vi "Main.vi"() -> ()   [LabVIEW 2017]
doc: "This Continuous Measurement sample project is based on the Queued Message Handler template.\n\nThe Event Handling Loop generates messages based on user interface actions.\n\nThe Message Handling Loop processes messages generated by the Event Handling Loop, or by other messages. There are also Acquisition and Logging message handling loop subVIs, and a chart updating loop."
uses:
  Settings/Settings.ctl
  Acquisition/Hardware Configuration.ctl
  Acquisition/Signal Type.ctl
  Logging/Logging Configuration.ctl
  controls/UI Data.ctl
  controls/UI State.ctl
  support/Message Queue/Enqueue Message (Single).vi
  support/Message Queue/Enqueue Message (Array).vi
  <vilib>/Utility/error.llb/Error Cluster From Error Code.vi
  <vilib>/ErrorRing/Error Ring.xnode
  Acquisition/Acquisition.lvlib
  Logging/Logging.lvlib
  Settings/Settings.lvlib
  support/User Event - Stop/User Event - Stop.lvlib
  support/Message Queue/Message Queue.lvlib
  Settings/Settings Dialog.vi
panel:
  out "Elapsed time":timestamp
  in  "Start waves":bool
  in  "Initialize wave maker":bool
  in  "Preview wave file":bool
  in  "Wave file":path
  in  "Testing time zero run [s]":dbl
  in  "Testing time [s]":dbl
  in  "Zero run?":bool
  in  "Stop":bool
  in  "Start":bool
  in  "Settings":bool
  out "Status":string
  in  "Exit":bool
  out "Waves preview":waveform(dbl)[](graph)
  out "Data":waveform(dbl)[](graph)
  # "Continuous Measurement Data Logger"
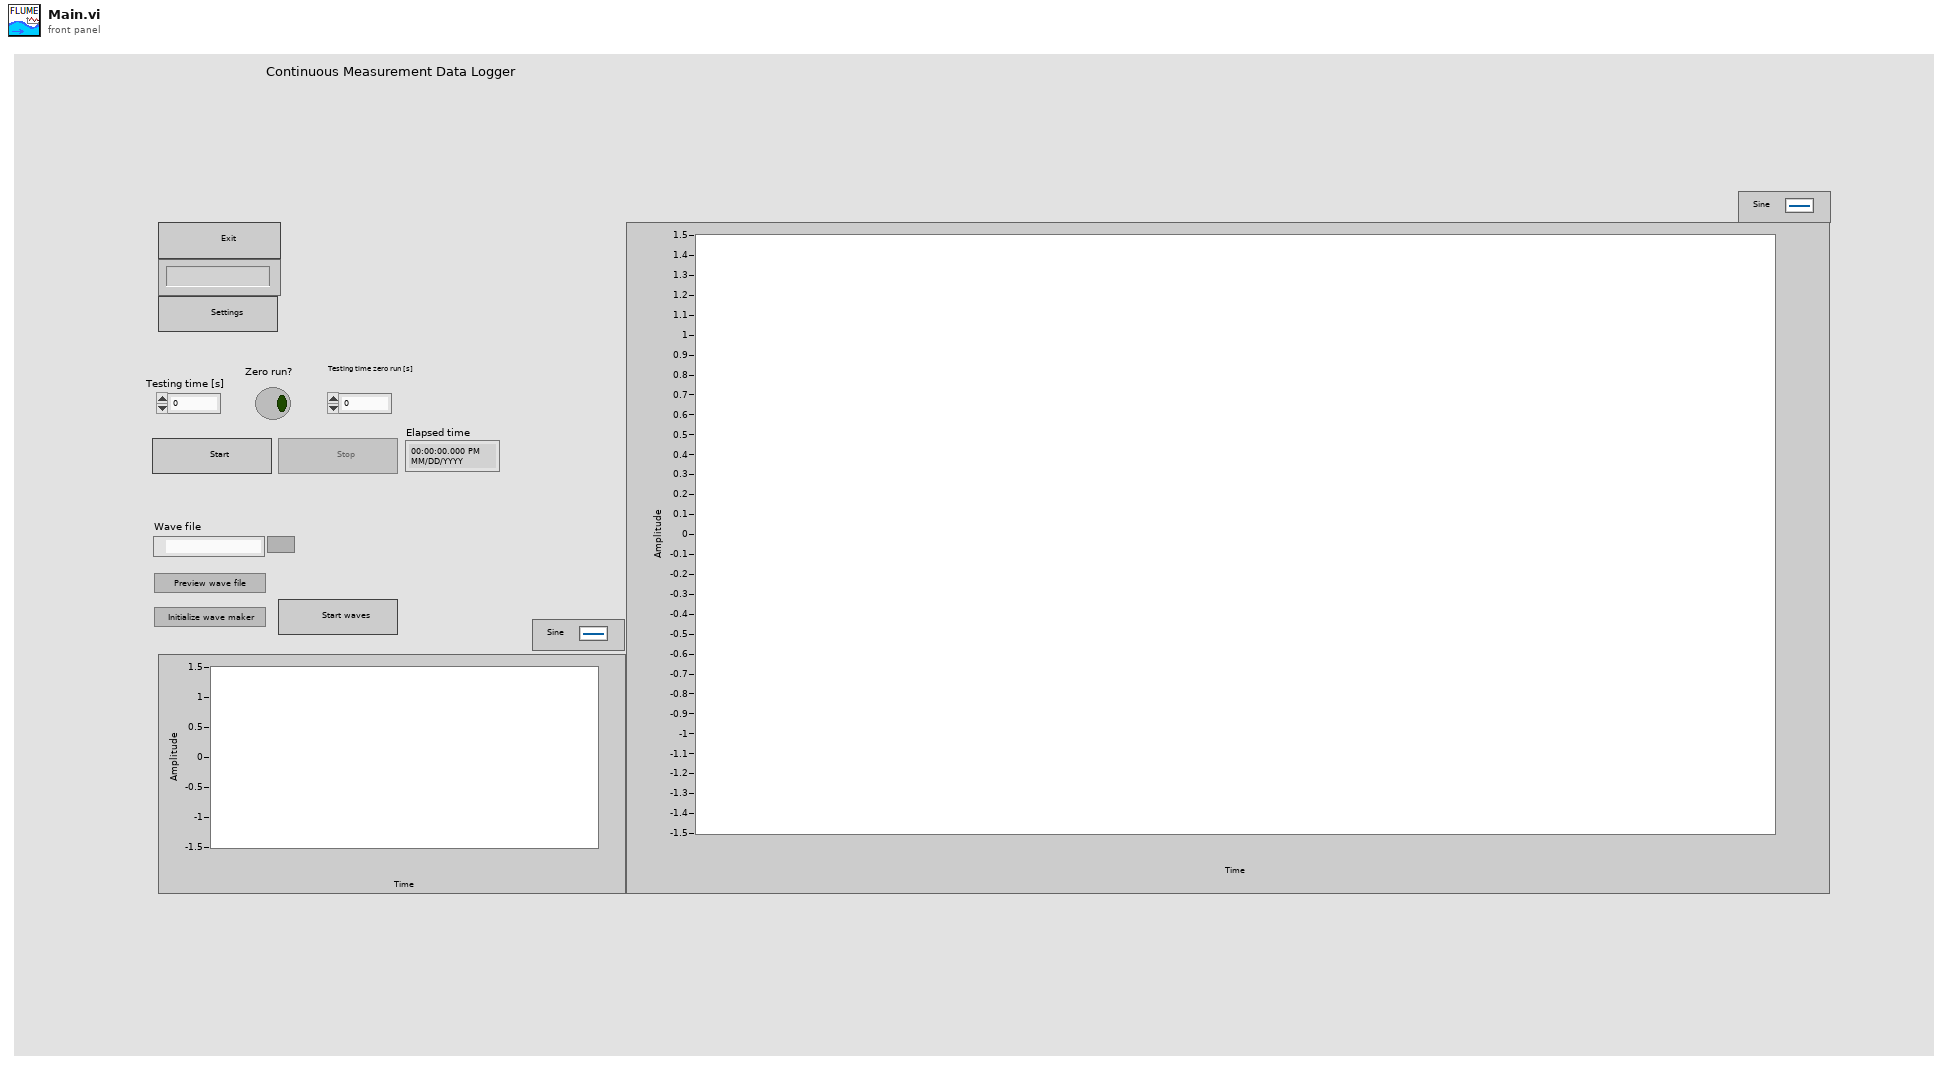
[diagram p1: front panel]
types:
  T1 = typedef "UI State.ctl" = enum16{"Idle", "Acquiring and Logging", "Waiting for Exit", "Waiting for Exit (Acq Stopped)", "Waiting for Exit (Log Stopped)", "Waiting for Stop", "Waiting for Stop (Acq Stopped)", "Waiting for Stop (Log Stopped)"}
  T2 = typedef "UI Data.ctl" = cluster{"Start Ref":refnum<vi>, "Stop Ref":refnum<vi>, "Settings Ref":refnum<vi>, "Exit Ref":refnum<vi>, "Status Ref":refnum<vi>, "Data Ref":refnum<vi>, "Start Waves Ref":refnum<vi>, "Wave Preview Ref":refnum<vi>, "Elapsed Time Ref":timestamp}
  T3 = typedef "Settings.lvlib/Settings.ctl" = cluster{"Hardware Configuration":T4, "Logging Configuration":T6}
  T4 = typedef "Acquisition.lvlib/Hardware Configuration.ctl" = cluster{"HW Refnum <Replace Me>":string, "Signal Type <Replace Me>":T5}
  T5 = typedef "Acquisition.lvlib/Signal Type.ctl" = enum16{"Sine Wave", "Square with Noise"}
  T6 = typedef "Logging.lvlib/Logging Configuration.ctl" = cluster{"Log File Base Path":path, "TDMS File Reference":refnum<k34>, "Log File Offsite Path":path, "Offsite storage?":bool, "Project code":string}
  T7 = typedef "Message Queue.lvlib/All Message Queues.ctl" = cluster{"UI":refnum<queue>, "Acquisition":refnum<queue>, "Logging":refnum<queue>}
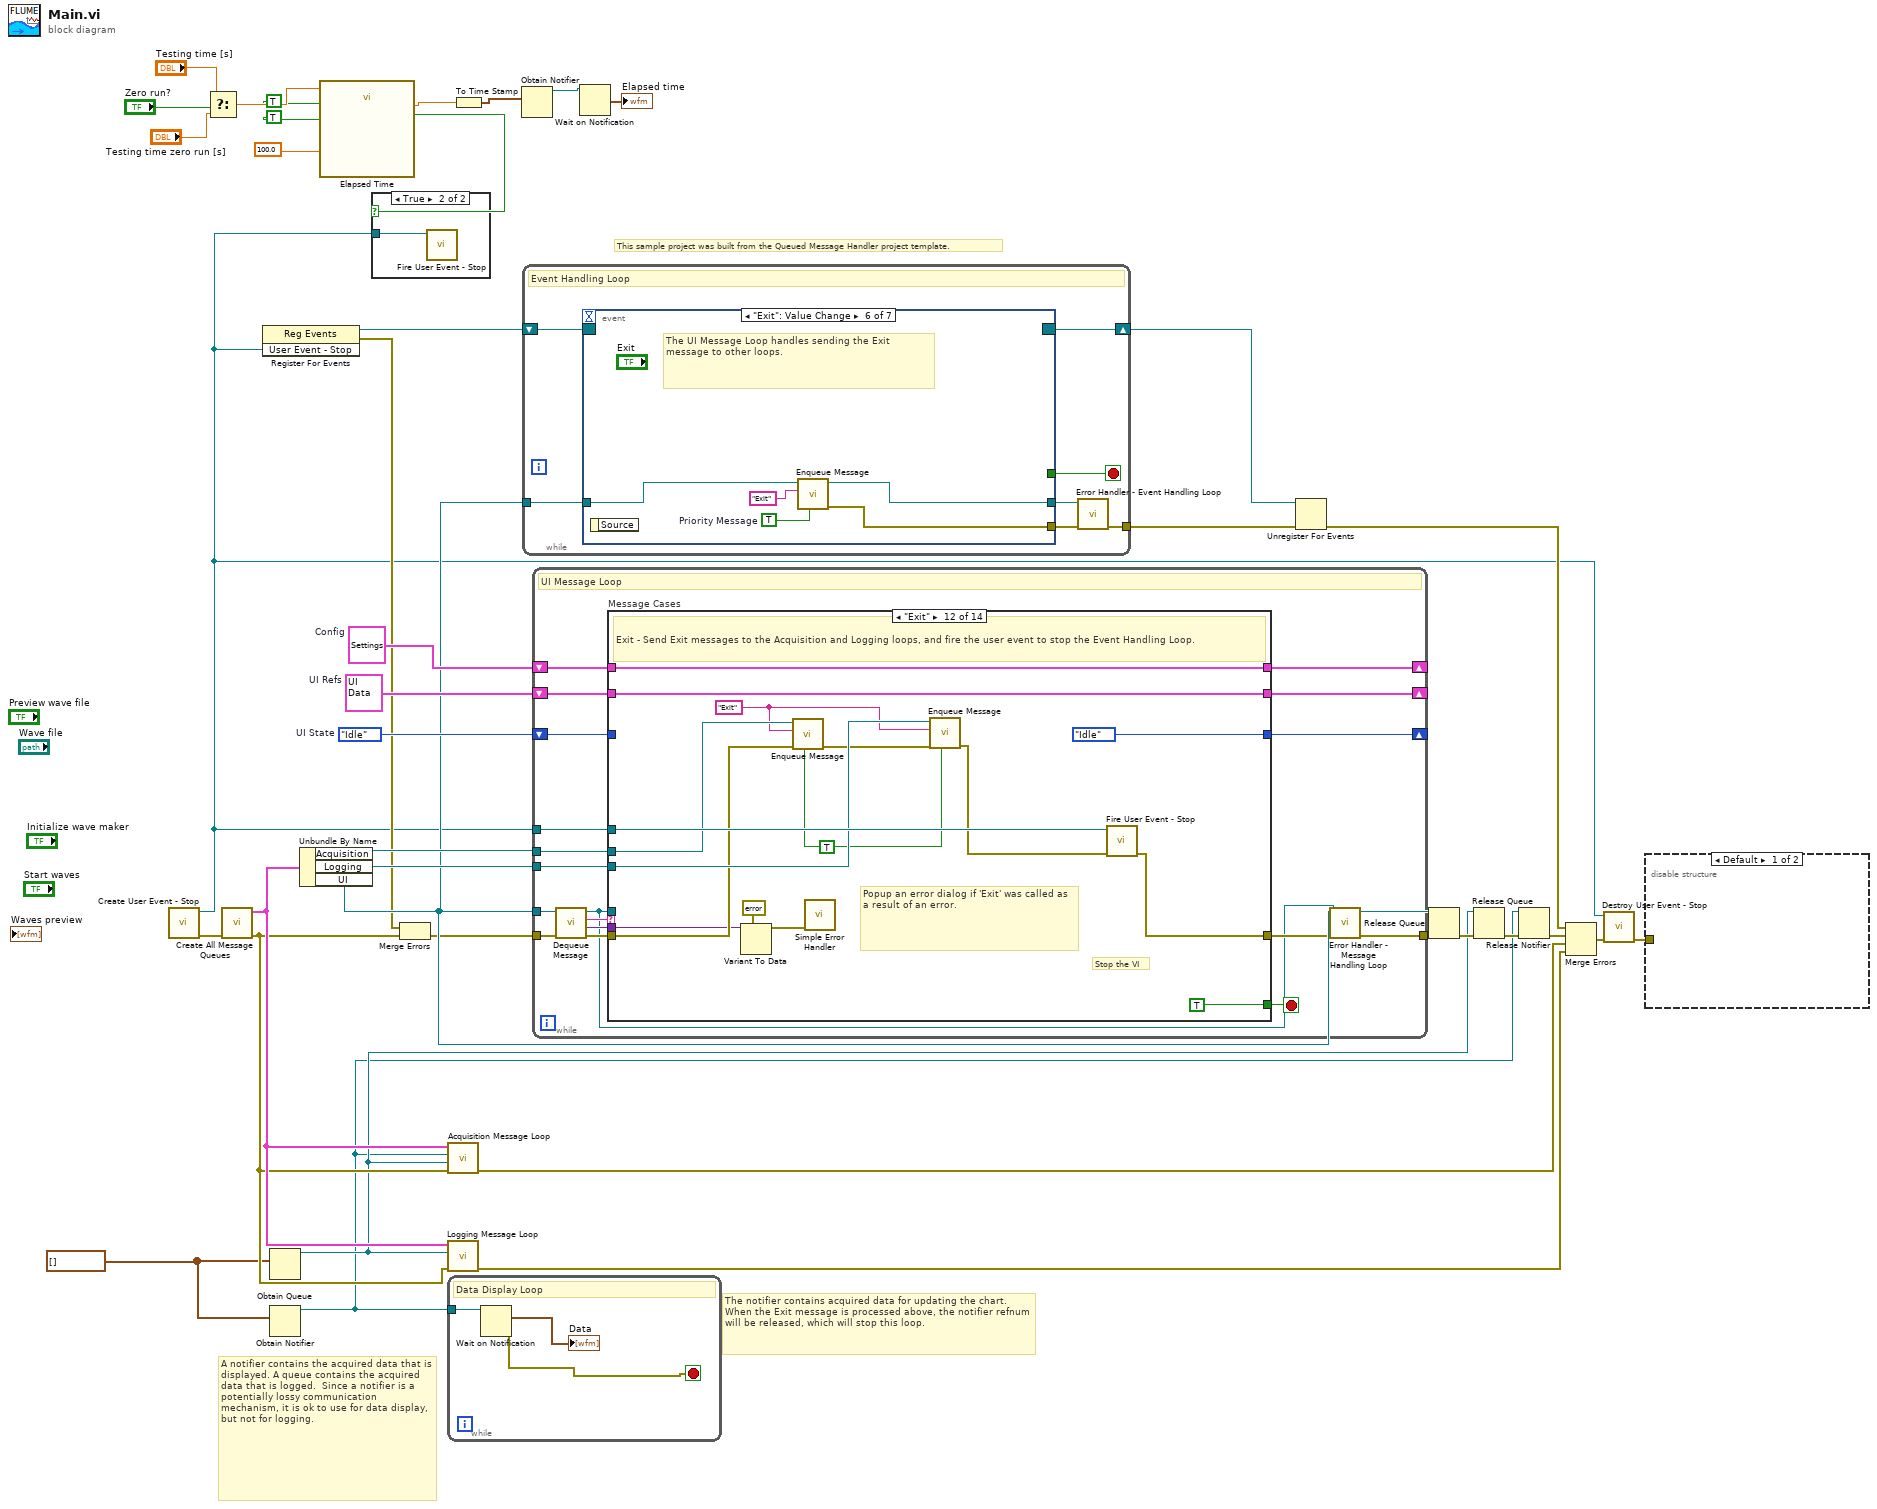
[diagram p0: block diagram]
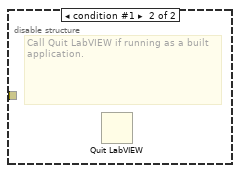
[diagram p3: hidden frame]
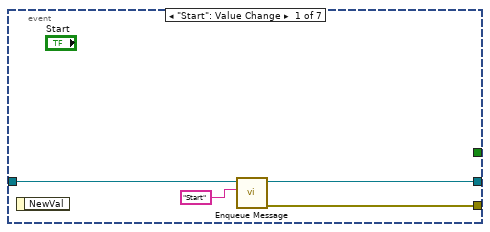
[diagram p4: hidden frame]
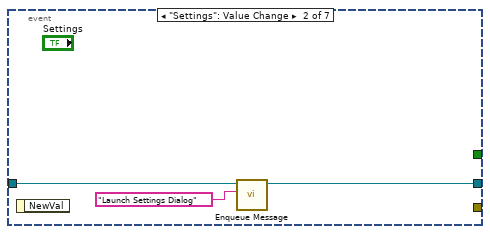
[diagram p5: hidden frame]
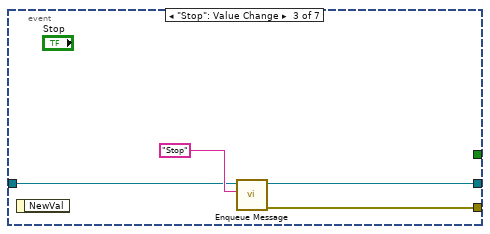
[diagram p6: hidden frame]
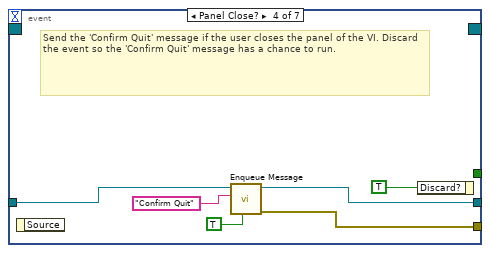
[diagram p7: hidden frame]
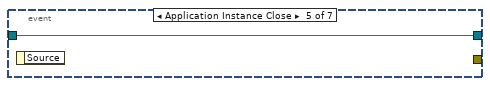
[diagram p8: hidden frame]
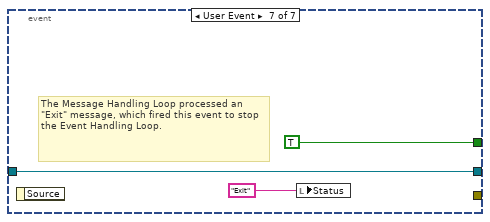
[diagram p9: hidden frame]
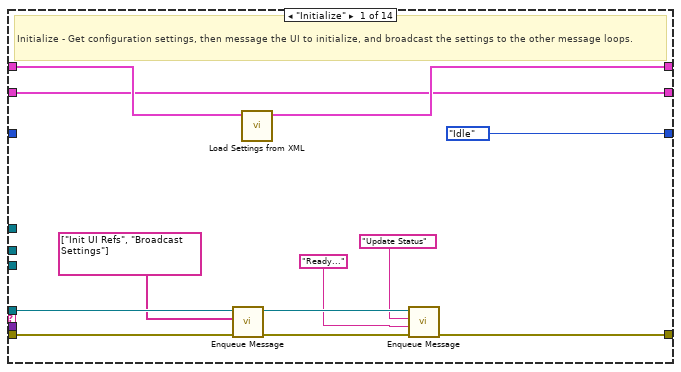
[diagram p10: hidden frame]
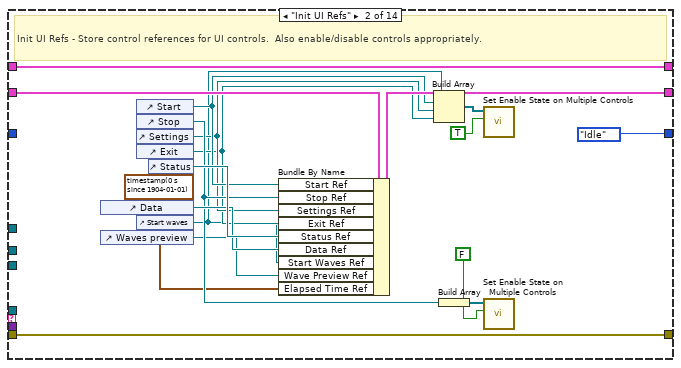
[diagram p11: hidden frame]
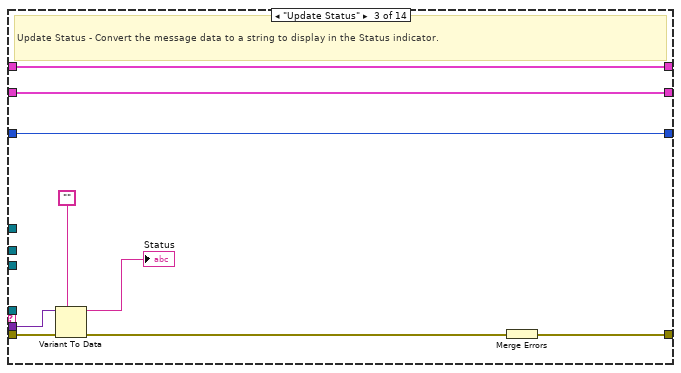
[diagram p12: hidden frame]
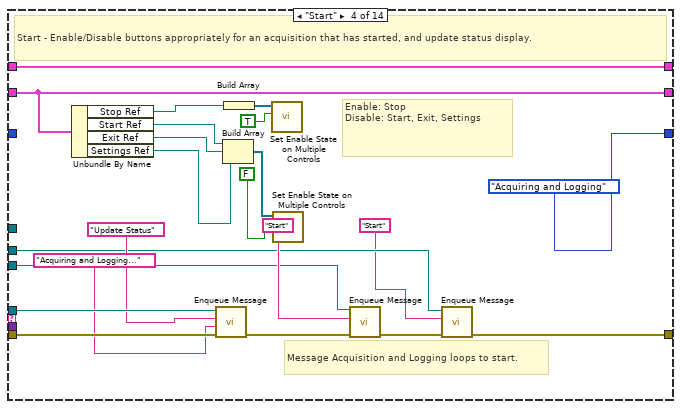
[diagram p13: hidden frame]
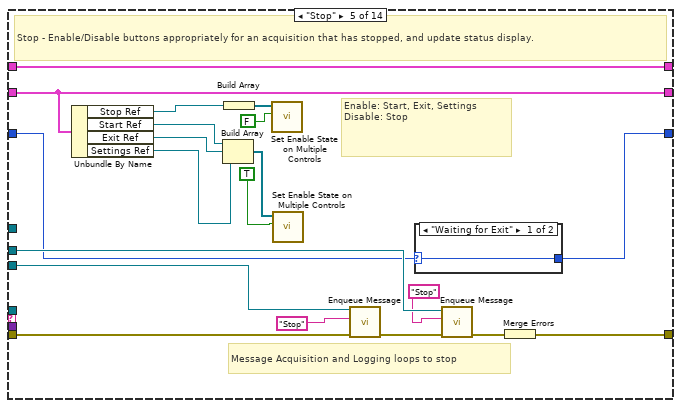
[diagram p14: hidden frame]
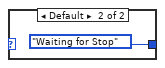
[diagram p15: hidden frame]
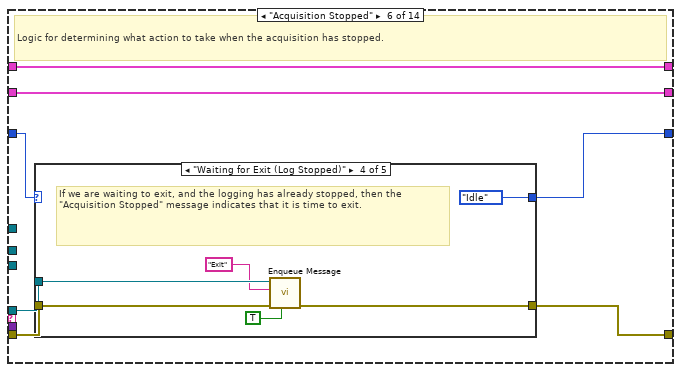
[diagram p16: hidden frame]
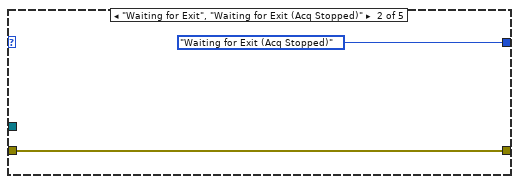
[diagram p18: hidden frame]
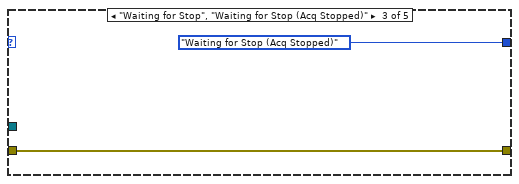
[diagram p19: hidden frame]
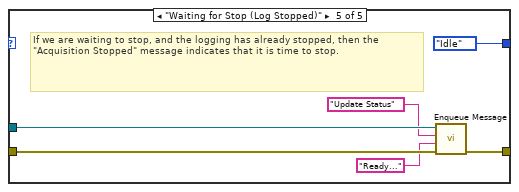
[diagram p20: hidden frame]
diagram:
  w26 = UI_State."Idle"  # UI State
  w17 = waveform(dbl)[] []
  w29 = T2 {"Start Ref"=refnum, "Stop Ref"=refnum, "Settings Ref"=refnum, "Exit Ref"=refnum, "Status Ref"=refnum, "Data Ref"=refnum, "Start Waves Ref"=refnum, "Wave Preview Ref"=refnum, "Elapsed Time Ref"=timestamp(0 s since 1904-01-01)}  # UI Refs
  w32 = T3 {"Hardware Configuration"={"HW Refnum <Replace Me>"="", "Signal Type <Replace Me>"=enum."Sine Wave"}, "Logging Configuration"={"Log File Base Path"=path "", "TDMS File Reference"=refnum, "Log File Offsite Path"=path "", "Offsite storage?"=FALSE, "Project code"=""}}  # Config
  # "This sample project was built from the Queued Message Handler project template."
  # "A notifier contains the acquired data that is displayed. A queue contains the acquired data that is logged.  Since a notifier is a potentially lossy communication mechanism, it is ok to use for data display, but not for logging."
  # "The notifier contains acquired data for updating the chart. When the Exit message is processed above, the notifier refnum will be released, which will stop this loop."
  n1 = call "Create User Event - Stop.vi"() -> ("error out"=w36:errorcluster, "User Event - Stop"=w1:refnum<user-event>)  [unwired: 10 in]
  n2 = Select(t="Testing time [s]", s="Zero run?", f="Testing time zero run [s]") -> (s? t:f=w10:dbl)
  n3 = call "Create All Message Queues.vi"("error in (no error)"=w36) -> ("error out"=w33:errorcluster, "Message Queues out"=w35:T7)  [unwired: 9 in]
  n4 = register-events(w1) -> (reference out=w16:refnum<event-registration>, error out=w14:errorcluster)  [unwired: 2 in]
  n5 = Obtain Queue(element data type=w17) -> (queue out=w19:refnum<queue>)  [unwired: 4 in, 2 out]
  n6 = Obtain Notifier(notification data type=w17) -> (notifier out=w18:refnum<notifier>)  [unwired: 3 in, 2 out]
  n7 = Unbundle By Name(w35) -> ("Acquisition"=w28:refnum<queue>, "Logging"=w27:refnum<queue>, "UI"=w24:refnum<queue>)
  n8 = call "Elapsed Time"("Time Target (s)"=w10, "Reset"=TRUE, "Auto Reset"=TRUE, "Set Start Time (s)"=100.0) -> ("Elapsed Time (s)"=w6:dbl, "Time has Elapsed"=w2:bool)  [unwired: 8 in, 6 out]
  n9 = case shown="True" w2 {
    tunnel: w1 -> [_ w40]
    frame False {
    }
    frame True {
      n10 = call "Fire User Event - Stop.vi"("User Event - Stop"=w40) -> ()  [unwired: 10 in, 1 out]
    }
  }
  n11 = Merge Errors(w14, w33) -> (w15:errorcluster)
  n12 = call "Acquisition Message Loop.vi"("error in (no error)"=w33, "Data Queue"=w19, "Data Notifier"=w18, "Message Queues"=w35) -> ("error out"=w37:errorcluster)  [unwired: 7 in]
  n13 = call "Logging Message Loop.vi"("error in (no error)"=w33, "Data Queue"=w19, "Message Queues"=w35) -> ("error out"=w34:errorcluster)  [unwired: 8 in]
  n14 = while "Data Display Loop" {
    tunnel: w18 -> [w43]
    stop <- w41 stop-if-true
    # "Data Display Loop"
    n15 = Wait on Notification(notifier=w43) -> (notification=→"Data":waveform(dbl)[], error out=w41:errorcluster)  [unwired: 3 in, 2 out]
  }
  n16 = To Time Stamp(1:w6) -> (0:w5:timestamp)
  n17 = Obtain Notifier(notification data type=w5) -> (notifier out=w3:refnum<notifier>)  [unwired: 3 in, 2 out]
  n18 = while {
    tunnel: w24 -> [w49]
    tunnel: [w46] -> w38
    shift-right: [w48] -> w30
    shift-left: w16 -> [w50]
    stop <- w47 stop-if-true
    # "Event Handling Loop"
    n19 = event shown="[5] \"Exit\": Value Change" {
      selector: w50 -> [_ _ _ _ _ _ _]
      dyn-events: [_ _ _ _ _ _ _] -> w48
      timeout: _ -> [_ _ _ _ _ _ _]
      tunnel: [_ _ _ _ _ _ TRUE ("Discard?")] -> w47
      tunnel: w49 -> [w54 w56 w60 w65 w68 w70 w74]
      tunnel: [w52 _ w59 w63 _ w73 _] -> w45
      tunnel: [w51 w55 w58 w64 w68 w69 w74] -> w44
      event "Start": Value Change {
        n20 = event-data() -> ()  [unwired: 1 in, 1 out]
        n21 = call-poly "Enqueue Message.vi"("Message"="Start", "Message Queue"=w54) -> ("error out"=w52:errorcluster, "dup Message Queue"=w51:refnum<queue>)  [unwired: 8 in]
      }
      event "Settings": Value Change {
        n22 = event-data() -> ()  [unwired: 1 in, 1 out]
        n23 = call-poly "Enqueue Message.vi"("Message"="Launch Settings Dialog", "Message Queue"=w56) -> ("dup Message Queue"=w55:refnum<queue>)  [unwired: 8 in, 1 out]
      }
      event "Stop": Value Change {
        n24 = event-data() -> ()  [unwired: 1 in, 1 out]
        n25 = call-poly "Enqueue Message.vi"("Message"="Stop", "Message Queue"=w60) -> ("error out"=w59:errorcluster, "dup Message Queue"=w58:refnum<queue>)  [unwired: 8 in]
      }
      event Panel Close? {
        # "Send the 'Confirm Quit' message if the user closes the panel of the VI. Discard the event so the 'Confirm Quit' message has a chance to run."
        n26 = event-data() -> ()  [unwired: 1 in, 1 out]
        n27 = call-poly "Enqueue Message.vi"("Priority Message? (F)"=TRUE, "Message"="Confirm Quit", "Message Queue"=w65) -> ("error out"=w63:errorcluster, "dup Message Queue"=w64:refnum<queue>)  [unwired: 7 in]
        n28 = event-data("Discard?"=TRUE) -> ()  [unwired: 1 in, 1 out]
      }
      event Application Instance Close {
        n29 = event-data() -> ()  [unwired: 1 in, 1 out]
      }
      event "Exit": Value Change {
        w71 = TRUE  # Priority Message
        # "The UI Message Loop handles sending the Exit message to other loops."
        n30 = event-data() -> ()  [unwired: 1 in, 1 out]
        n31 = call-poly "Enqueue Message.vi"("Priority Message? (F)"=w71, "Message"="Exit", "Message Queue"=w70) -> ("error out"=w73:errorcluster, "dup Message Queue"=w69:refnum<queue>)  [unwired: 7 in]
      }
      event User Event {
        # "The Message Handling Loop processed an \"Exit\" message, which fired this event to stop the Event Handling Loop."
        n32 = event-data() -> ()  [unwired: 1 in, 1 out]
        n33 = local write "Status"("Exit" ("Exit String")) -> ()
      }
    }
    n34 = call "Error Handler - Event Handling Loop.vi"("error in (no error)"=w45, "Message Queue"=w44) -> ("dup error in"=w46:errorcluster)  [unwired: 8 in, 1 out]
  }
  n35 = while {
    tunnel: w24 -> [w88]
    tunnel: w1 -> [w93]
    shift-right: [w87] -> _
    shift-left: w32 -> [w86]
    shift-right: [w84] -> _
    shift-left: w29 -> [w85]
    tunnel: w28 -> [w83]
    tunnel: w27 -> [w82]
    shift-right: [w77] -> _
    shift-left: w26 -> [w78]
    tunnel: w15 -> [w92]
    tunnel: [w81] -> w39
    stop <- w94 stop-if-true
    # "UI Message Loop"
    n36 = call "Dequeue Message.vi"("error in (no error)"=w92, "Message Queue"=w88) -> ("error out"=w91:errorcluster, "Message Data"=w89:variant, "Message"=w90:string, "dup Message Queue"=w79:refnum<queue>)  [unwired: 6 in]
    n37 = case "Message Cases" shown="\"Exit\"" w90 {
      selector: w90 -> [_ _ _ _ _ _ _ _ _ _ _ _ _ w313]
      tunnel: w79 -> [w98 _ _ w155 _ w180 w205 _ w245 _ w266 _ _ _]
      tunnel: w91 -> [w97 w124 w132 w154 w174 w181 w206 w236 w247 w254 w265 w295 w311 _]
      tunnel: [w102 w124 w133 w137 w175 w178 w203 w239 w241 w257 w264 w304 w310 w312] -> w80
      tunnel: [_ _ _ _ _ _ _ _ _ _ _ TRUE _ _] -> w94
      tunnel: w89 -> [_ _ w131 _ _ _ _ _ _ w258 _ w293 _ _]
      tunnel: w93 -> [_ _ _ _ _ _ _ _ _ _ _ w305 _ _]
      tunnel: [w105 w123 w125 w153 w173 w184 w209 w230 w240 w262 w269 w303 w309 w316] -> w87
      tunnel: w86 -> [w106 w123 w125 w153 w173 w184 w209 w230 w248 w262 w269 w303 w309 w316]
      tunnel: w85 -> [w99 w122 w127 w150 w172 w183 w208 w234 w243 w261 w268 w302 w308 w315]
      tunnel: [w99 w119 w127 w150 w172 w183 w208 w234 w243 w261 w268 w302 w308 w315] -> w84
      tunnel: w83 -> [_ _ _ w136 w159 _ _ w233 _ _ _ w301 _ _]
      tunnel: w82 -> [_ _ _ w139 w162 _ _ w232 _ _ _ w300 _ _]
      tunnel: w78 -> [_ _ w126 _ w156 w182 w207 w231 w242 w256 w267 _ w307 w314]
      tunnel: [UI_State."Idle" ("UI State") UI_State."Idle" ("UI State") w126 UI_State."Acquiring and Logging" ("UI State") w157 w179 w204 w231 w242 w256 w263 UI_State."Idle" ("UI State") w307 w314] -> w77
      frame "Initialize" {
        # "Initialize - Get configuration settings, then message the UI to initialize, and broadcast the settings to the other message loops."
        n38 = call-poly "Enqueue Message.vi"("error in (no error)"=w97, "Message Array"=string[] ["Init UI Refs", "Broadcast Settings"], "Message Queue"=w98) -> ("error out"=w104:errorcluster, "dup Message Queue"=w103:refnum<queue>)  [unwired: 7 in]
        n39 = call "Load Settings from XML.vi"("Settings in"=w106) -> ("Settings out"=w105:T3)  [unwired: 9 in, 1 out]
        n40 = call-poly "Enqueue Message.vi"("error in (no error)"=w104, "Message Data"="Ready..." ("Ready..."), "Message"="Update Status", "Message Queue"=w103) -> ("error out"=w102:errorcluster)  [unwired: 6 in, 1 out]
      }
      frame "Init UI Refs" {
        # "Init UI Refs - Store control references for UI controls.  Also enable/disable controls appropriately."
        n41 = control-ref of="Data"() -> (w120:refnum<vi>)
        n42 = control-ref of="Waves preview"() -> (w109:refnum<vi>)
        n43 = control-ref of="Start"() -> (w113:refnum<vi>)
        n44 = control-ref of="Stop"() -> (w114:refnum<vi>)
        n45 = control-ref of="Settings"() -> (w112:refnum<vi>)
        n46 = control-ref of="Exit"() -> (w111:refnum<vi>)
        n47 = control-ref of="Start waves"() -> (w107:refnum<vi>)
        n48 = control-ref of="Status"() -> (w121:refnum<vi>)
        n49 = Bundle By Name(cluster=w122, "Start Ref"=w113, "Stop Ref"=w114, "Settings Ref"=w112, "Exit Ref"=w111, "Status Ref"=w121, "Data Ref"=w120, "Start Waves Ref"=w107, "Wave Preview Ref"=w109, "Elapsed Time Ref"=timestamp(0 s since 1904-01-01)) -> (w119:T2)
        n50 = Build Array(w107, w113, w112, w111) -> (w117:refnum<vi>[])
        n51 = Build Array(w114) -> (w116:refnum<vi>[])
        n52 = call "Set Enable State on Multiple Controls.vi"("Enable?"=TRUE, "Controls"=w117) -> ()  [unwired: 10 in]
        n53 = call "Set Enable State on Multiple Controls.vi"("Enable?"=FALSE, "Controls"=w116) -> ()  [unwired: 10 in]
      }
      frame "Update Status" {
        # "Update Status - Convert the message data to a string to display in the Status indicator."
        n54 = Variant To Data(error in=w132, type="", Variant=w131) -> (data=→"Status":string, error out=w129:errorcluster)
        n55 = Merge Errors(w129) -> (w133:errorcluster)
      }
      frame "Start" {
        # "Message Acquisition and Logging loops to start."
        # "Enable: Stop\nDisable: Start, Exit, Settings"
        # "Start - Enable/Disable buttons appropriately for an acquisition that has started, and update status display."
        n56 = Unbundle By Name(w150) -> ("Stop Ref"=w145:refnum<vi>, "Start Ref"=w144:refnum<vi>, "Exit Ref"=w143:refnum<vi>, "Settings Ref"=w142:refnum<vi>)
        n57 = call-poly "Enqueue Message.vi"("error in (no error)"=w154, "Message Data"="Acquiring and Logging..." ("Acquiring and Logging..."), "Message"="Update Status", "Message Queue"=w155) -> ("error out"=w141:errorcluster)  [unwired: 6 in, 1 out]
        n58 = Build Array(w144, w143, w142) -> (w148:refnum<vi>[])
        n59 = Build Array(w145) -> (w147:refnum<vi>[])
        n60 = call "Set Enable State on Multiple Controls.vi"("Enable?"=TRUE, "Controls"=w147) -> ()  [unwired: 10 in]
        n61 = call "Set Enable State on Multiple Controls.vi"("Enable?"=FALSE, "Controls"=w148) -> ()  [unwired: 10 in]
        n62 = call-poly "Enqueue Message.vi"("error in (no error)"=w141, "Message"="Start", "Message Queue"=w139) -> ("error out"=w138:errorcluster)  [unwired: 7 in, 1 out]
        n63 = call-poly "Enqueue Message.vi"("error in (no error)"=w138, "Message"="Start", "Message Queue"=w136) -> ("error out"=w137:errorcluster)  [unwired: 7 in, 1 out]
      }
      frame "Stop" {
        # "Message Acquisition and Logging loops to stop"
        # "Enable: Start, Exit, Settings\nDisable: Stop"
        # "Stop - Enable/Disable buttons appropriately for an acquisition that has stopped, and update status display."
        n64 = Unbundle By Name(w172) -> ("Stop Ref"=w167:refnum<vi>, "Start Ref"=w166:refnum<vi>, "Exit Ref"=w165:refnum<vi>, "Settings Ref"=w164:refnum<vi>)
        n65 = Build Array(w166, w165, w164) -> (w170:refnum<vi>[])
        n66 = Build Array(w167) -> (w169:refnum<vi>[])
        n67 = call "Set Enable State on Multiple Controls.vi"("Enable?"=FALSE, "Controls"=w169) -> ()  [unwired: 10 in]
        n68 = call "Set Enable State on Multiple Controls.vi"("Enable?"=TRUE, "Controls"=w170) -> ()  [unwired: 10 in]
        n69 = call-poly "Enqueue Message.vi"("error in (no error)"=w174, "Message"="Stop", "Message Queue"=w162) -> ("error out"=w161:errorcluster)  [unwired: 7 in, 1 out]
        n70 = case shown="\"Waiting for Exit\"" w156 {
          selector: w156 -> [w176 _]
          tunnel: [w176 UI_State."Waiting for Stop" ("UI State")] -> w157
          frame "Waiting for Exit" {
          }
          frame Default {
          }
        }
        n71 = call-poly "Enqueue Message.vi"("error in (no error)"=w161, "Message"="Stop", "Message Queue"=w159) -> ("error out"=w160:errorcluster)  [unwired: 7 in, 1 out]
        n72 = Merge Errors(w160) -> (w175:errorcluster)
      }
      frame "Acquisition Stopped" {
        # "Logic for determining what action to take when the acquisition has stopped."
        n73 = case shown="\"Waiting for Exit (Log Stopped)\"" w182 {
          selector: w182 -> [w186 _ _ _ _]
          tunnel: w181 -> [w185 w188 w190 w196 w202]
          tunnel: w180 -> [_ _ _ w194 w199]
          tunnel: [w186 UI_State."Waiting for Exit (Acq Stopped)" ("UI State") UI_State."Waiting for Stop (Acq Stopped)" ("UI State") UI_State."Idle" ("UI State") UI_State."Idle" ("UI State")] -> w179
          tunnel: [w185 w188 w190 w195 w200] -> w178
          frame Default {
          }
          frame "Waiting for Exit", "Waiting for Exit (Acq Stopped)" {
          }
          frame "Waiting for Stop", "Waiting for Stop (Acq Stopped)" {
          }
          frame "Waiting for Exit (Log Stopped)" {
            # "If we are waiting to exit, and the logging has already stopped, then the \"Acquisition Stopped\" message indicates that it is time to exit."
            n74 = call-poly "Enqueue Message.vi"("Priority Message? (F)"=TRUE, "error in (no error)"=w196, "Message"="Exit", "Message Queue"=w194) -> ("error out"=w195:errorcluster)  [unwired: 6 in, 1 out]
          }
          frame "Waiting for Stop (Log Stopped)" {
            # "If we are waiting to stop, and the logging has already stopped, then the \"Acquisition Stopped\" message indicates that it is time to stop."
            n75 = call-poly "Enqueue Message.vi"("error in (no error)"=w202, "Message Data"="Ready..." ("Ready..."), "Message"="Update Status", "Message Queue"=w199) -> ("error out"=w200:errorcluster)  [unwired: 6 in, 1 out]
          }
        }
      }
      frame "Logging Stopped" {
        # "Logic for determining what action to take when the logging has stopped."
        n76 = case shown="\"Waiting for Stop (Acq Stopped)\"" w207 {
          selector: w207 -> [w211 _ _ _ _]
          tunnel: w206 -> [w210 w213 w215 w221 w224]
          tunnel: w205 -> [_ _ _ w219 w223]
          tunnel: [w211 UI_State."Waiting for Exit (Log Stopped)" ("UI State") UI_State."Waiting for Stop (Log Stopped)" ("UI State") UI_State."Idle" ("UI State") UI_State."Idle" ("UI State")] -> w204
          tunnel: [w210 w213 w215 w220 w222] -> w203
          frame Default {
          }
          frame "Waiting for Exit", "Waiting for Exit (Log Stopped)" {
          }
          frame "Waiting for Stop", "Waiting for Stop (Log Stopped)" {
          }
          frame "Waiting for Exit (Acq Stopped)" {
            # "If we are waiting to exit, and the acquisition has already stopped, then the \"Logging Stopped\" message indicates that it is time to exit."
            n77 = call-poly "Enqueue Message.vi"("Priority Message? (F)"=TRUE, "error in (no error)"=w221, "Message"="Exit", "Message Queue"=w219) -> ("error out"=w220:errorcluster)  [unwired: 6 in, 1 out]
          }
          frame "Waiting for Stop (Acq Stopped)" {
            # "If we are waiting to stop, and the acquisition has already stopped, then the \"Logging Stopped\" message indicates that it is time to stop."
            n78 = call-poly "Enqueue Message.vi"("error in (no error)"=w224, "Message Data"="Ready..." ("Ready..."), "Message"="Update Status", "Message Queue"=w223) -> ("error out"=w222:errorcluster)  [unwired: 6 in, 1 out]
          }
        }
      }
      frame "Broadcast settings" {
        w235 = "Update Settings" ("Message")
        # "Broadcast settings - Send the 'Update Settings' message to the Logging and Acquisition message loops."
        n79 = Unbundle By Name(w230) -> ("Hardware Configuration"=w228:T4, "Logging Configuration"=w229:T6)
        n80 = call-poly "Enqueue Message.vi"("Message Data"=w228, "Message"=w235, "Message Queue"=w233) -> ("error out"=w238:errorcluster)  [unwired: 7 in, 1 out]
        n81 = call-poly "Enqueue Message.vi"("error in (no error)"=w238, "Message Data"=w229, "Message"=w235, "Message Queue"=w232) -> ("error out"=w237:errorcluster)  [unwired: 6 in, 1 out]
        n82 = Merge Errors(w237, w236) -> (w239:errorcluster)
      }
      frame "Launch Settings Dialog" {
        # "Launch Settings Dialog - Launch the Settings Dialog when the user clicks the 'Settings' button."
        n83 = call-by-ref "?"("error in (no error)"=w247, "Settings in"=w248) -> ("error out"=w244:errorcluster, "Cancelled?"=w246:bool, "Settings out"=w240:T3)  [unwired: 8 in, 3 out]
        n84 = case shown="False" w246 {
          tunnel: w245 -> [w252 _]
          tunnel: w244 -> [w251 w253]
          tunnel: [w250 w253] -> w241
          frame False {
            n85 = call-poly "Enqueue Message.vi"("error in (no error)"=w251, "Message"="Broadcast Settings", "Message Queue"=w252) -> ("error out"=w250:errorcluster)  [unwired: 7 in, 1 out]
          }
          frame True {
          }
        }
      }
      frame "Error" {
        # "Error - Display an error dialog. This message is sent by the \"Error Handler\" VIs at the end of other loops in this application."
        n86 = Variant To Data(error in=w254, type=errorcluster {"status"=FALSE, "code"=0, "source"=""} ("error constant"), Variant=w258) -> (data=w255:errorcluster, error out=w259:errorcluster)
        n87 = call <vilib>:"Simple Error Handler.vi"("error in (no error)"=w255) -> ()  [unwired: 4 in, 5 out]
        n88 = Merge Errors(w259) -> (w257:errorcluster)
      }
      frame "Confirm Quit" {
        # "Confirm Quit - Message that can confirm whether or not the user wants to exit the application."
        n89 = case shown="\"Acquiring and Logging\"" w267 {
          tunnel: w266 -> [w275 w279]
          tunnel: w265 -> [w274 w278]
          tunnel: [w273 w277] -> w264
          tunnel: [UI_State."Idle" ("UI State") w276] -> w263
          frame Default {
            # "If 'Confirm Quit' comes in while the system is idle, there is no need for a confirmation message."
            n90 = call-poly "Enqueue Message.vi"("Priority Message? (F)"=TRUE, "error in (no error)"=w274, "Message"="Exit", "Message Queue"=w275) -> ("error out"=w273:errorcluster)  [unwired: 6 in, 1 out]
          }
          frame "Acquiring and Logging" {
            n91 = Two Button Dialog(message="Are you sure you want to quit while the acquisition is running?" ("Confirm Quit Message"), 1:"No" ("No"), 2:"Yes" ("Yes")) -> (T button?=w280:bool)
            n92 = case shown="True" w280 {
              tunnel: w279 -> [_ w289]
              tunnel: w278 -> [w285 w290]
              tunnel: [w285 w288] -> w277
              tunnel: [UI_State."Acquiring and Logging" ("UI State") UI_State."Waiting for Exit" ("UI State")] -> w276
              frame False {
                # "User did not want to quit."
              }
              frame True {
                n93 = call-poly "Enqueue Message.vi"("error in (no error)"=w290, "Message"="Stop", "Message Queue"=w289) -> ("error out"=w288:errorcluster)  [unwired: 7 in, 1 out]
              }
            }
          }
        }
      }
      frame "Exit" {
        w291 = TRUE ("Priority Message? (F)")
        w297 = "Exit" ("Message")
        # "Popup an error dialog if 'Exit' was called as a result of an error."
        # "Stop the VI"
        # "Exit - Send Exit messages to the Acquisition and Logging loops, and fire the user event to stop the Event Handling Loop."
        n94 = Variant To Data(type=errorcluster {"status"=FALSE, "code"=0, "source"=""} ("error constant"), Variant=w293) -> (data=w292:errorcluster)  [unwired: 1 in, 1 out]
        n95 = call-poly "Enqueue Message.vi"("Priority Message? (F)"=w291, "error in (no error)"=w295, "Message"=w297, "Message Queue"=w301) -> ("error out"=w298:errorcluster)  [unwired: 6 in, 1 out]
        n96 = call <vilib>:"Simple Error Handler.vi"("error in (no error)"=w292) -> ()  [unwired: 4 in, 5 out]
        n97 = call-poly "Enqueue Message.vi"("Priority Message? (F)"=w291, "error in (no error)"=w298, "Message"=w297, "Message Queue"=w300) -> ("error out"=w296:errorcluster)  [unwired: 6 in, 1 out]
        n98 = call "Fire User Event - Stop.vi"("error in (no error)"=w296, "User Event - Stop"=w305) -> ("error out"=w304:errorcluster)  [unwired: 9 in]
      }
      frame "---Copy This Frame---" {
        # "Duplicate this frame when creating new messages.  Change this comment in the duplicated frame to describe this message."
        n99 = Merge Errors(w311) -> (w310:errorcluster)
      }
      frame Default {
        # "'Default' case only runs if there is a message that isn't defined in any of the other cases.  Output a programming error."
        n100 = xnode "Error Ring"("parameter 0"=w313) -> ("error out"=w312:errorcluster)
      }
    }
    n101 = call "Error Handler - Message Handling Loop.vi"("error in (no error)"=w80, "Message Queue"=w79) -> ("dup error in"=w81:errorcluster)  [unwired: 8 in, 1 out]
  }
  n102 = Wait on Notification(notifier=w3) -> (notification=→"Elapsed time":timestamp)  [unwired: 3 in, 3 out]
  n103 = Unregister For Events(event registration refnum=w30, error in=w38) -> (error out=w31:errorcluster)
  n104 = Release Queue(queue=w24, error in (no error)=w39) -> (error out=w22:errorcluster)  [unwired: 1 in, 2 out]
  n105 = Release Queue(queue=w19, error in (no error)=w22) -> (error out=w21:errorcluster)  [unwired: 1 in, 2 out]
  n106 = Release Notifier(notifier=w18, error in (no error)=w21) -> (error out=w20:errorcluster)  [unwired: 1 in, 2 out]
  n107 = Merge Errors(w31, w20, w37, w34) -> (w25:errorcluster)
  n108 = call "Destroy User Event - Stop.vi"("error in (no error)"=w25, "User Event - Stop"=w1) -> ("error out"=w23:errorcluster)  [unwired: 9 in]
  n109 = disable-structure shown="Default" {
    disable-tunnel: w23 -> [_ _]
    frame condition #0 (active) {
    }
    frame condition #1 {
      # "Call Quit LabVIEW if running as a built application."
      n110 = Quit LabVIEW() -> ()  [unwired: 1 in]
    }
  }
